vi "Fluke 5080 AC DC Current Calibrator.vi"() -> ()   [LabVIEW 2012]
doc: "This example shows how to configure the calibrator to ac/dc current voltage output mode."
uses:
  <instrlib>/Fluke 5080/Fluke 5080.lvlib
panel:
  in  "Current (1.0 A)":dbl=0.5
  in  "Output Post Binding (0: AUX)":i32(ring) items=["AUX", "20A"]
  in  "Inductive Compensation Enabled (T: Enabled)":bool=TRUE
  in  "Serial Configuration":T1={"Baud Rate"=9600, "Parity"=0, "Data Bits"=8, "Stop Bits"=10, "Flow Control"=0} {"Flow Control" items=["None", "XON/XOFF", "RTS/CTS", "XON/XOFF & RTS/CTS", "DTR/DSR", "XON/XOFF & DTR/DSR"]; "Stop Bits" items=["1.0"=10, "1.5"=15, "2.0"=20]; "Data Bits" items=["7"=7, "8"=8]; "Parity" items=["None", "Odd", "Even", "Mark", "Space"]; "Baud Rate" items=["300"=300, "600"=600, "1200"=1200, "2400"=2400, "4800"=4800, "9600"=9600, "19200"=19200]}
  in  "VISA resource name":refnum<visa-resource-name>
  in  "Frequency (50.0 Hertz)":dbl=50.0
  in  "Phase (0.0 Degrees)":dbl
  in  "Output Type (0: DC Volts)":i32(ring)=3 items=["DC Volts", "AC Volts", "DC Current", "AC Current", "DC Power", "AC Power", "Dual DC Volts", "Dual AC Volts", "Resistance"]
  in  "Earth Ground Enabled (T: Enabled)":bool=TRUE
  # "(c) 2010 National Instruments.  ALL RIGHTS RESERVED."
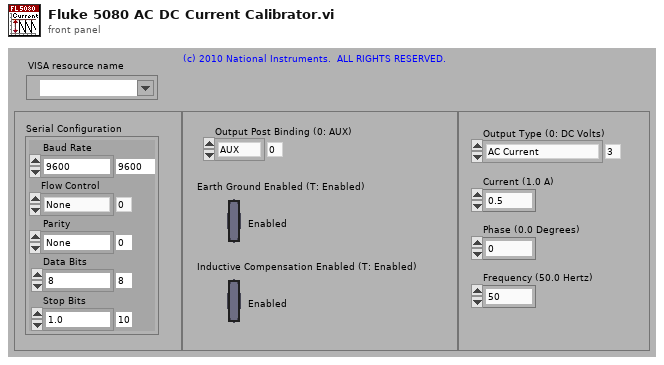
[diagram p1: front panel]
types:
  T1 = cluster{"Baud Rate":u32, "Parity":u16, "Data Bits":u16, "Stop Bits":u16, "Flow Control":u16}
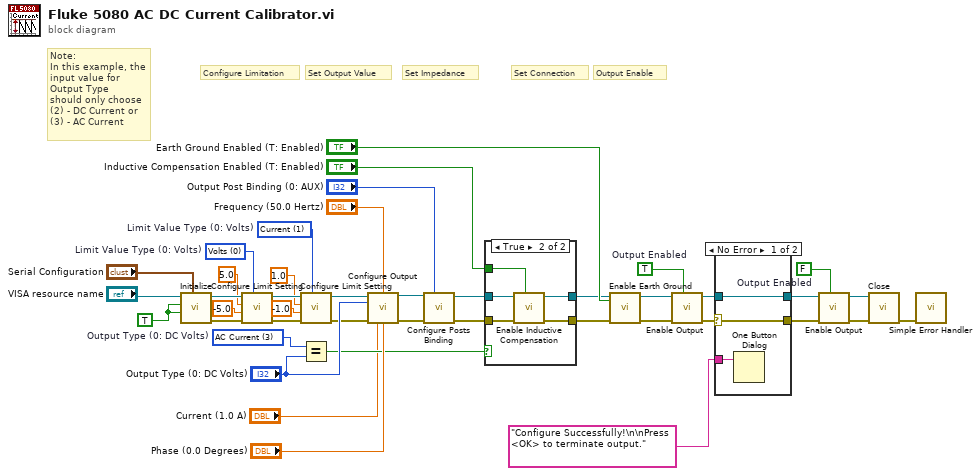
[diagram p0: block diagram]
diagram:
  w5 = 0 items=["Volts", "Current"]  # Limit Value Type (0: Volts)
  w6 = 1 items=["Volts", "Current"]  # Limit Value Type (0: Volts)
  w18 = FALSE  # Output Enabled
  w19 = TRUE  # Output Enabled
  w29 = 3 items=["DC Volts", "AC Volts", "DC Current", "AC Current", "DC Power", "AC Power", "Dual DC Volts", "Dual AC Volts", "Resistance"]  # Output Type (0: DC Volts)
  w42 = TRUE ("Reset (True)")
  # "Set Connection"
  # "Note:\nIn this example, the \ninput value for \nOutput Type\nshould only choose \n(2) - DC Current or \n(3) - AC Current"
  # "Output Enable"
  # "Set Impedance"
  # "Set Output Value"
  # "Configure Limitation"
  n1 = call <instrlib>:"Initialize.vi"("Serial Configuration"="Serial Configuration", "Reset (True)"=w42, "ID Query (True)"=w42, "VISA resource name"="VISA resource name") -> ("error out"=w40:errorcluster, "VISA resource name out"=w39:refnum<visa-resource-name>)  [unwired: 1 in, 5 out]
  n2 = call <instrlib>:"Configure Limit Setting.vi"("Limit Value Type (0: Volts)"=w5, "error in (no error)"=w40, "- Limit Value (-5)"=-5.0, "+ Limit Value (5)"=5.0, "VISA resource name"=w39) -> ("error out"=w8:errorcluster, "VISA resource name out"=w10:refnum<visa-resource-name>)  [unwired: 5 out]
  n3 = call <instrlib>:"Configure Limit Setting.vi"("Limit Value Type (0: Volts)"=w6, "error in (no error)"=w8, "- Limit Value (-5)"=-1.0, "+ Limit Value (5)"=1.0, "VISA resource name"=w10) -> ("error out"=w7:errorcluster, "VISA resource name out"=w9:refnum<visa-resource-name>)  [unwired: 5 out]
  n4 = Equal?(x=w29, y="Output Type (0: DC Volts)") -> (x = y?=w27:bool)
  n5 = call <instrlib>:"Configure Output.vi"("VISA resource name"=w9, "Frequency (50.0 Hertz)"="Frequency (50.0 Hertz)", "Output Type (0: DC Volts)"="Output Type (0: DC Volts)", "error in (no error)"=w7, "Current (1.0 A)"="Current (1.0 A)", "Phase (0.0 Degrees)"="Phase (0.0 Degrees)") -> ("VISA resource name out"=w25:refnum<visa-resource-name>, "error out"=w22:errorcluster)  [unwired: 4 in, 4 out]
  n6 = call <instrlib>:"Configure Posts Binding.vi"("error in (no error)"=w22, "Output Post Binding (0: AUX)"="Output Post Binding (0: AUX)", "VISA resource name"=w25) -> ("error out"=w23:errorcluster, "VISA resource name out"=w24:refnum<visa-resource-name>)  [unwired: 7 out]
  n7 = case shown="True" w27 {
    tunnel: [w44 w49] -> w33
    tunnel: [w43 w48] -> w32
    tunnel: w23 -> [w43 w47]
    tunnel: w24 -> [w44 w46]
    tunnel: "Inductive Compensation Enabled (T: Enabled)" -> [_ w45]
    frame False {
    }
    frame True {
      n8 = call <instrlib>:"Enable Inductive Compensation.vi"("Inductive Compensation Enabled (T: Enabled)"=w45, "error in (no error)"=w47, "VISA resource name"=w46) -> ("error out"=w48:errorcluster, "VISA resource name out"=w49:refnum<visa-resource-name>)  [unwired: 7 out]
    }
  }
  n9 = call <instrlib>:"Enable Earth Ground.vi"("Earth Ground Enabled (T: Enabled)"="Earth Ground Enabled (T: Enabled)", "error in (no error)"=w32, "VISA resource name"=w33) -> ("error out"=w30:errorcluster, "VISA resource name out"=w31:refnum<visa-resource-name>)  [unwired: 7 out]
  n10 = call <instrlib>:"Enable Output.vi"("Output Enabled (T: Enable)"=w19, "error in (no error)"=w30, "VISA resource name"=w31) -> ("error out"=w16:errorcluster, "VISA resource name out"=w17:refnum<visa-resource-name>)  [unwired: 7 out]
  n11 = case shown="No Error" w16 {
    selector: w16 -> [w51 w53]
    tunnel: "Configure Successfully!\n\nPress <OK> to terminate output." ("message") -> [w52 _]
    tunnel: [w51 w53] -> w13
    tunnel: [w50 w54] -> w14
    tunnel: w17 -> [w50 w54]
    frame No Error {
      n12 = One Button Dialog(message=w52) -> ()  [unwired: 2 out]
    }
    frame Error {
    }
  }
  n13 = call <instrlib>:"Enable Output.vi"("Output Enabled (T: Enable)"=w18, "error in (no error)"=w13, "VISA resource name"=w14) -> ("error out"=w11:errorcluster, "VISA resource name out"=w12:refnum<visa-resource-name>)  [unwired: 7 out]
  n14 = call <instrlib>:"Close.vi"("error in (no error)"=w11, "VISA resource name"=w12) -> ("error out"=w36:errorcluster)  [unwired: 9 out]
  n15 = call <vilib>:"Simple Error Handler.vi"("error in (no error)"=w36) -> ()  [unwired: 1 in, 8 out]
